vi "strip extension.vi"(1 "Path":path) -> (0 "stripped extension":string)   [LabVIEW 2015]
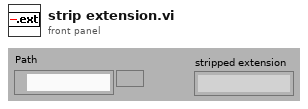
[diagram p1: front panel]
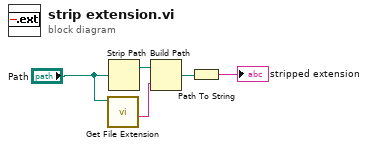
[diagram p0: block diagram]
diagram:
  n1 = call <vilib>:"Get File Extension.vi"("file"="Path") -> ("filename without extension"=w3:string)  [unwired: 6 in, 4 out]
  n2 = Strip Path(path="Path") -> (stripped path=w4:path)  [unwired: 1 out]
  n3 = Build Path(base path=w4, name or relative path=w3) -> (appended path=w2:path)
  n4 = Path To String(path=w2) -> (string=→"stripped extension":string)
